vi "Routing_Data.vi"(7 "Table Name":string, 8 "error in (no error)":errorcluster, 11 "Refnum in":T1) -> (0 "error out":errorcluster, 1 "Pokeyoke":bool[](array[boolean]), 2 "Routing":bool[](array[boolean]), 3 "Refnum out":T1, 4 "OperationCode":string[](array[string]), 6 "MachineCode":string[](array[string]))   [LabVIEW 2020]
uses:
  <vilib>/addons/database/Connection.llb/Conn ObjectReference.ctl
  <vilib>/addons/database/NI_Database_API.lvlib
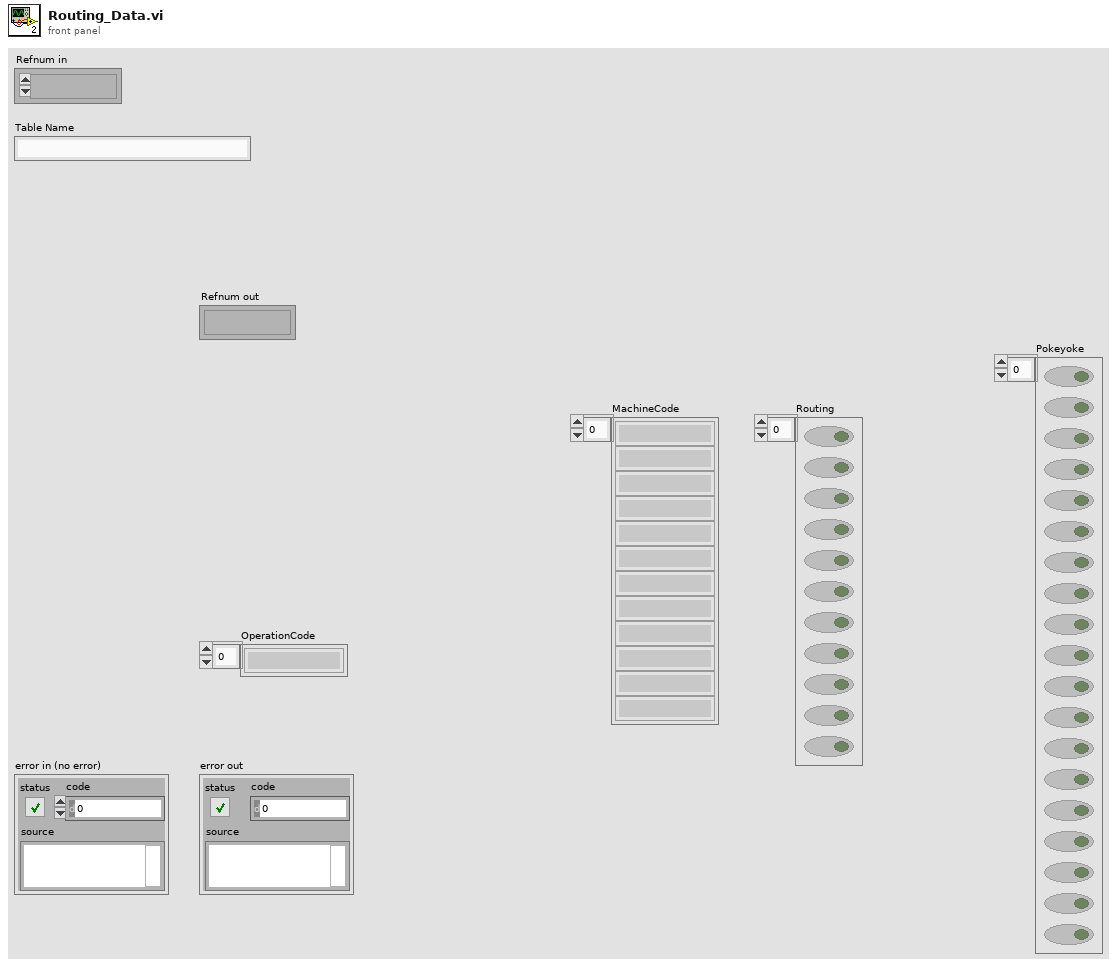
[diagram p1: front panel]
types:
  T1 = typedef "NI_Database_API.lvlib/Conn ObjectReference.ctl" = refnum<k1>
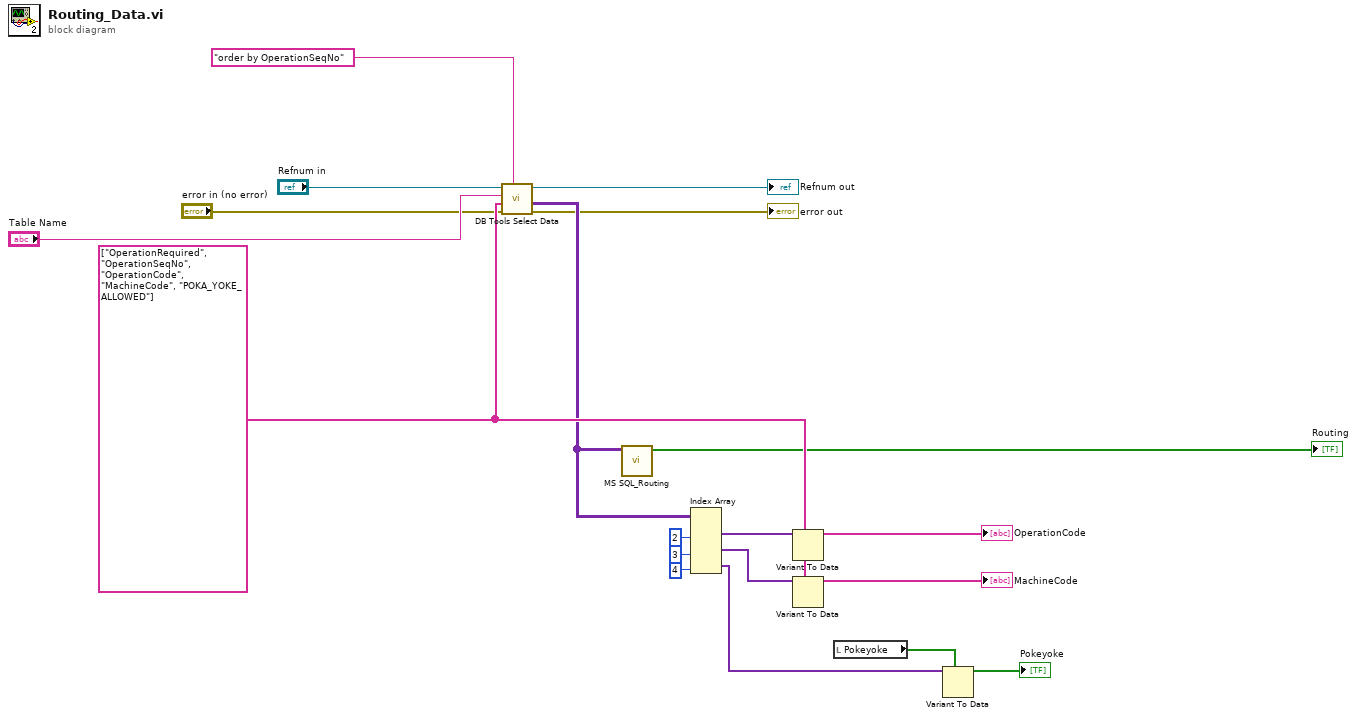
[diagram p0: block diagram]
diagram:
  w16 = string[] ["OperationRequired", "OperationSeqNo", "OperationCode", "MachineCode", "POKA_YOKE_ALLOWED"] ("columns")
  n1 = call <vilib>:"DB Tools Select Data.vi"("condition"="order by OperationSeqNo", "error in (no error)"="error in (no error)", "columns"=w16, "table"="Table Name", "connection reference"="Refnum in") -> ("error out"=→"error out":errorcluster, "data"=w13:variant[][], "connection reference out"=→"Refnum out":T1)  [unwired: 1 in]
  n2 = call "MS SQL_Routing.vi"("data"=w13) -> ("Array"=→"Routing":bool[])  [unwired: 10 in]
  n3 = Index Array(array=w13, index (col) #1=2 ("disabled index (col)"), index (col) #2=3 ("index (col)"), index (col) #3=4 ("index (col)")) -> (element #1=w14:variant[], element #2=w15:variant[], element #3=w7:variant[])  [unwired: 3 in]
  n4 = Variant To Data(type=w16, Variant=w14) -> (data=→"OperationCode":string[])  [unwired: 1 in, 1 out]
  n5 = Variant To Data(type=w16, Variant=w15) -> (data=→"MachineCode":string[])  [unwired: 1 in, 1 out]
  n6 = local read "Pokeyoke"() -> (w5:bool[])
  n7 = Variant To Data(type=w5, Variant=w7) -> (data=→"Pokeyoke":bool[])  [unwired: 1 in, 1 out]
